vi "Find Native Path.vi"() -> (3 "path":path)   [LabVIEW 2025, in "WebView2.lvlib" / "WebView2 Control.lvclass"]
uses:
  WebView2 Control.lvclass
  <vilib>/Utility/LVLibp/NI_PackedLibraryUtility.lvlib
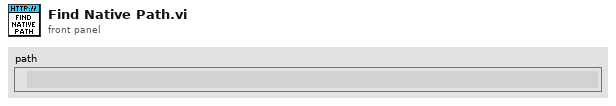
[diagram p1: front panel]
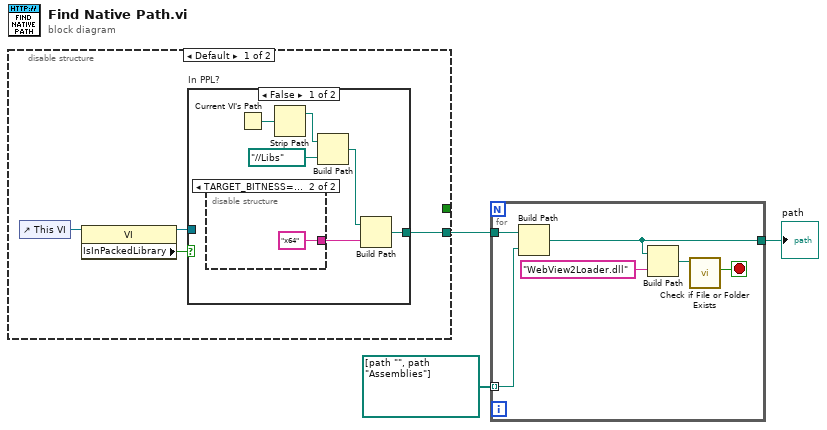
[diagram p0: block diagram]
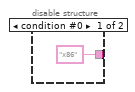
[diagram p2: hidden frame]
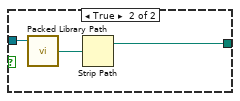
[diagram p3: hidden frame]
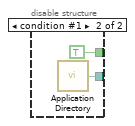
[diagram p4: hidden frame]
diagram:
  n1 = disable-structure shown="Default" {
    disable-tunnel: [_ TRUE] -> _
    disable-tunnel: [w4 w19] -> w2
    frame condition #0 (active) {
      n2 = control-ref of="This VI"() -> (w7:refnum<vi>)
      n3 = property class="VI"(reference=w7) -> (reference out=w5:refnum<vi>, "IsInPackedLibrary"=w6:bool)  [unwired: 1 in, 1 out]
      n4 = case "In PPL?" shown="False" w6 {
        tunnel: w5 -> [_ w17]
        tunnel: [w8 w16] -> w4
        frame False {
          n5 = disable-structure shown="TARGET_BITNESS==64" {
            disable-tunnel: ["x86" "x64"] -> w11
            frame condition #0 {
            }
            frame condition #1 (active) {
            }
          }
          n6 = Current VI's Path() -> (path=w13:path)
          n7 = Strip Path(path=w13) -> (stripped path=w12:path)  [unwired: 1 out]
          n8 = Build Path(base path=w12, name or relative path=path "../../Libs") -> (appended path=w10:path)
          n9 = Build Path(base path=w10, name or relative path=w11) -> (appended path=w8:path)
        }
        frame True {
          n10 = call <vilib>:"Packed Library Path.vi"("vi reference"=w17) -> ("packed library path"=w18:path)  [unwired: 2 in, 2 out]
          n11 = Strip Path(path=w18) -> (stripped path=w16:path)  [unwired: 1 out]
        }
      }
    }
    frame condition #1 {
      n12 = call <vilib>:"Application Directory.vi"() -> ("Application Directory"=w19:path)
    }
  }
  n13 = for {
    tunnel: w2 -> [w26]
    tunnel: path[] [path "", path "Assemblies"] ("name or relative path") -> [w25] mode=indexing
    tunnel: [w21] -> w3
    stop <- w22 stop-if-true
    n14 = Build Path(base path=w26, name or relative path=w25) -> (appended path=w21:path)
    n15 = Build Path(base path=w21, name or relative path="WebView2Loader.dll") -> (appended path=w23:path)
    n16 = call <vilib>:"Check if File or Folder Exists.vi"("path"=w23) -> ("file or folder exists?"=w22:bool)  [unwired: 8 in, 2 out]
  }
  "path" <- w3
